vi "Request Synchronous Data (Variant).vi"(6 "Ignore Past Updates? (F)":bool, 7 "Timeout In ms (-1)":i32=-1, 8 "error in (no error)":errorcluster, 9 "Type":variant, 10 "Datum Name":string, 11 "IModel In":refnum<class "IModel.lvclass">) -> (0 "error out":errorcluster, 1 "timed out?":bool, 2 "Data":variant, 4 "Publication Time":timestamp)   [LabVIEW 2015, in "IModel.lvlib" / "IModel.lvclass"]
doc: "<License>\nCopyright © 2017 Composed Systems, LLC | All rights reserved\nwww.composed.io\n\nAuthor: Ethan Stern <ethan.stern@composed.io>\n\nThis software is provided \"AS IS\" WITHOUT WARRANTIES, either express or implied, AND IS FOR EDUCATIONAL PURPOSES ONLY.\n</License>"
uses:
  IModel.lvclass
  Transport/QueueTransport/QueueTransport.lvclass/QueueTransport.ctl
  <vilib>/ActorFramework/Actor/Actor.lvclass/Actor.ctl
  <vilib>/ActorFramework/Message Enqueuer/Message Enqueuer.lvclass/Message Enqueuer.ctl
  IModel.lvclass/IModel.ctl
  SubscriptionPolicy/OneShotSubscription/OneShotSubscription.lvclass/OneShotSubscription.ctl
  AbstractMessages/PreAddressedMsg/PreAddressedMsg.lvclass/PreAddressedMsg.ctl
  IMediator/IMediator Messages/Subscribe Msg/Subscribe Msg.lvclass/Subscribe Msg.ctl
  <vilib>/ActorFramework/Actor/Read Self Enqueuer.vi
  <vilib>/ActorFramework/Message Enqueuer/Enqueue.vi
  AbstractMessages/PreAddressedMsg/Read Return Address.vi
  <vilib>/ActorFramework/Message Enqueuer/Init from Existing Queue.vi
  <vilib>/ActorFramework/Message Priority Queue/Priority Enqueue.vi
  <vilib>/Utility/error.llb/Error Cluster From Error Code.vi
  <vilib>/ActorFramework/Message Enqueuer/Message Enqueuer.lvclass
  SubscriptionPolicy/OneShotSubscription/OneShotSubscription.lvclass
  Transport/QueueTransport/QueueTransport.lvclass
  IMediator/SubscriptionRequest/SubscriptionRequest.lvclass
  IMediator/ISubscriptionPolicy/ISubscriptionPolicy.lvclass
  IMediator/IMediator Messages/Subscribe Msg/Subscribe Msg.lvclass
  IObserver/IObserver/IObserver.lvclass
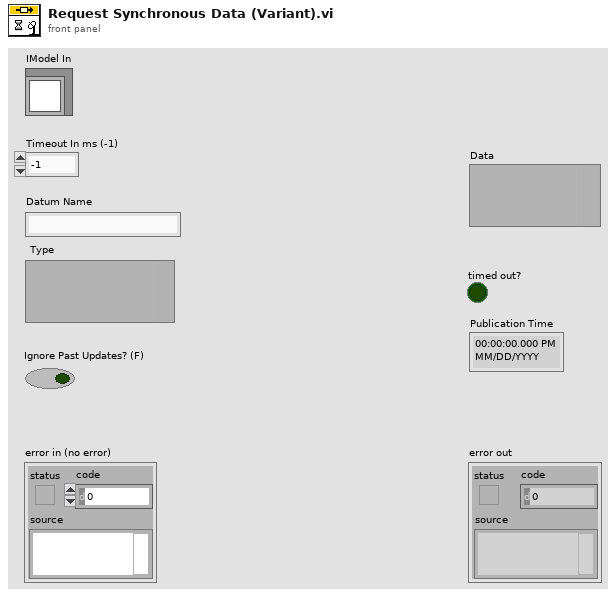
[diagram p1: front panel]
types:
  T1 = typedef "IMediator.lvlib/ISubscriptionPolicy.lvclass/ISubscriptionPolicy Reference.ctl" = refnum<data-value>
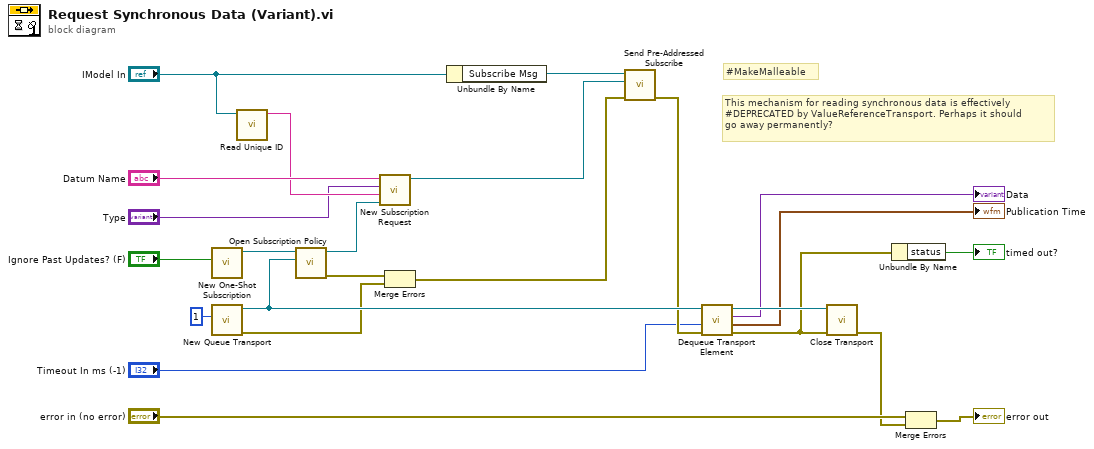
[diagram p0: block diagram]
diagram:
  # "#MakeMalleable"
  # "This mechanism for reading synchronous data is effectively\n#DEPRECATED by ValueReferenceTransport. Perhaps it should\ngo away permanently?"
  n1 = call "New One-Shot Subscription.vi"("Ignore Past Updates? (F)"="Ignore Past Updates? (F)") -> ("OneShotSubscription Out"=w17:refnum<class "OneShotSubscription.lvclass">)  [unwired: 10 in]
  n2 = call "New Queue Transport.vi"("Max Queue Size (-1)"=1 ("Max Queue Size (-1, unlimited)")) -> ("error out"=w9:errorcluster, "QueueTransport"=w11:refnum<class "QueueTransport.lvclass">)  [unwired: 9 in]
  n3 = call "Read Unique ID.vi"("IObserver In"="IModel In") -> ("Unique ID"=w19:string)  [unwired: 10 in]
  n4 = call "Open Subscription Policy.vi"("Transport"=w11, "SubscriptionPolicy"=w17) -> ("error out"=w12:errorcluster, "Subscription Policy"=w20:T1)  [unwired: 8 in]
  n5 = call "New Subscription Request.vi"("Subscription Policy"=w20, "Subscriber ID"=w19, "Type"="Type", "Datum Name"="Datum Name") -> ("SubscriptionRequest"=w13:refnum<class "SubscriptionRequest.lvclass">)  [unwired: 7 in]
  n6 = Merge Errors(w12, w9) -> (w10:errorcluster)
  n7 = Unbundle By Name("IModel In") -> ("Subscribe Msg"=w14:refnum<class "Subscribe Msg.lvclass">)
  n8 = call "Send Pre-Addressed Subscribe.vi"("error in (no error)"=w10, "Subscription Request"=w13, "Subscribe Msg"=w14) -> ("error out"=w8:errorcluster)  [unwired: 8 in]
  n9 = call "Dequeue Transport Element.vi"("error in (no error)"=w8, "Timeout In ms (-1)"="Timeout In ms (-1)", "QueueTransport in"=w11) -> ("error out"=w1:errorcluster, "Publication Time"=→"Publication Time":timestamp, "Data"=→"Data":variant, "QueueTransport out"=w24:refnum<class "QueueTransport.lvclass">)  [unwired: 5 in]
  n10 = call-dynamic "Close Transport.vi"("error in (no error)"=w1, "QueueTransport in"=w24) -> ("error out"=w3:errorcluster)  [unwired: 9 in]
  n11 = Unbundle By Name(w1) -> ("status"=→"timed out?":bool)
  n12 = Merge Errors("error in (no error)", w3) -> (→"error out":errorcluster)
